vi "main_0510.vi"() -> ()   [LabVIEW 2018]
uses:
  <vilib>/Platform/TimedLoop/XDataNode/timing_clust.ctl
  <vilib>/Platform/TimedLoop/XDataNode/nitl_modes.ctl
  <vilib>/Platform/TimedLoop/XDataNode/wakeup.ctl
  <vilib>/FPGAPlugInAG/myRIO-1900/niLvFpga_Open_myRIO-1900.vi
  <vilib>/rvi/interface/common/dynamic/niFpgaDynamicAddResources.vi
  <vilib>/Utility/error.llb/Error Cluster From Error Code.vi
  <vilib>/rvi/errors/niLvFpgaAdjustHostInterfaceError.vi
  <vilib>/rvi/interface/nirviOpenFPGA/nirviOpenFPGA.xnode
  FPGA Bitfiles/Dentalrobot_FPGATarget_FPGADentalroboto_PTkoih3chUc.lvbitx
  FPGA/FPGA_myRIO.vi
  <vilib>/rvi/interface/nirviReadWriteControl/nirviReadWriteControl.xnode
  <vilib>/Platform/TimedLoop/XDataNode/XDataNode.xnode
  <vilib>/Platform/TimedLoop/XDataNode/XDNodeRunTimeDep.lvlib
  <vilib>/rvi/interface/Simulation/niFpgaSimulationCallBeginRW.vi
  NiFpgaLv.dll
panel:
  in  "Voltage Detect":bool
  in  "temp":i32
  in  "inverse(degree)":i32=90
  in  "limit_mV":u16=2000
  out "Finished Late":dbl
  in  "DIR4":bool
  out "Position4":i32
  in  "Reset 4":bool
  in  "STBY4":bool
  in  "ENA4":bool
  in  "CH4 DC":fxp<+,32,0>
  in  "RPM":string(combo)="150"
  in  "step":u32 step=2
  in  "Dir":bool=TRUE
  out "Voltage Detection (mV)":u16(graph)=459
  out "storeDC":fxp<+,32,0>[](array[numeric])
  in  "Inv":bool
  out "mV":u16
  in  "OK Button":bool
  out "position":i32[](array[numeric])
  out "Signal":bool[](array[boolean])
  out "Over Range":bool
  in  "stop":bool
  in  "Position":dbl step=1.0
  # "Servor"
  # "Stepper"
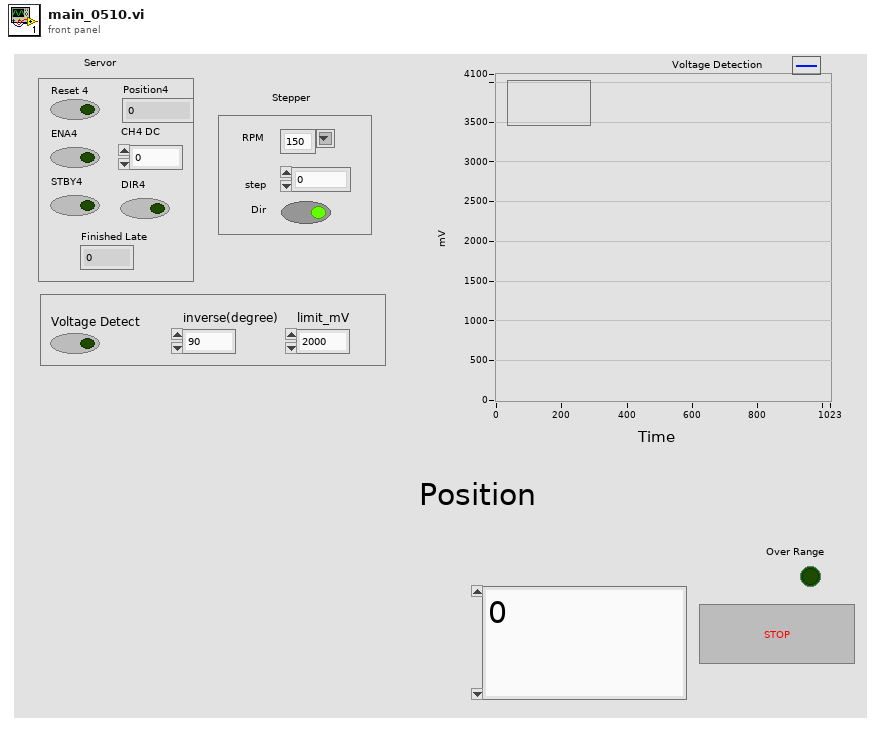
[diagram p1: front panel]
types:
  T1 = typedef "XDNodeRunTimeDep.lvlib/timing_clust.ctl" = cluster{"Expected End [f-1]":u64, "Actual End [f-1]":u64, "Finished Late? [f-1]":bool, "Expected End [i-1]":u64, "Actual End [i-1]":u64, "Finished Late? [i-1]":bool, "Expected Start [i]":u64, "Actual Start [i]":u64, "Expected Start [f]":u64, "Actual Start [f]":u64, "Source Name":string, "Structure Name":string, "Period":i64, "Deadline":i64, "Offset":i64, "Start":i64, "Priority":i32, "Timeout":i32, "Mode":T2, "Wakeup Reason":T3, "Error":errorcluster, "Source Type":string, "Secondary Source Type":string, "Global End Time":u64, "Global Start Time":u64, "Frame Duration":u64, "Iteration Duration":u64, "Assigned CPU":i32, "I/O Scan Engine Mode":u32}
  T2 = typedef "XDNodeRunTimeDep.lvlib/nitl_modes.ctl" = enum32{"No Change", "Process missed periods, maintain original phase", "Discard missed periods, maintain original phase", "Process missed periods, ignore original phase", "Discard missed periods, ignore original phase"}
  T3 = typedef "XDNodeRunTimeDep.lvlib/wakeup.ctl" = enum32{"Normal", "Aborted", "Asynchronous wakeup", "Timing source error", "Timed loop error", "Timeout"}
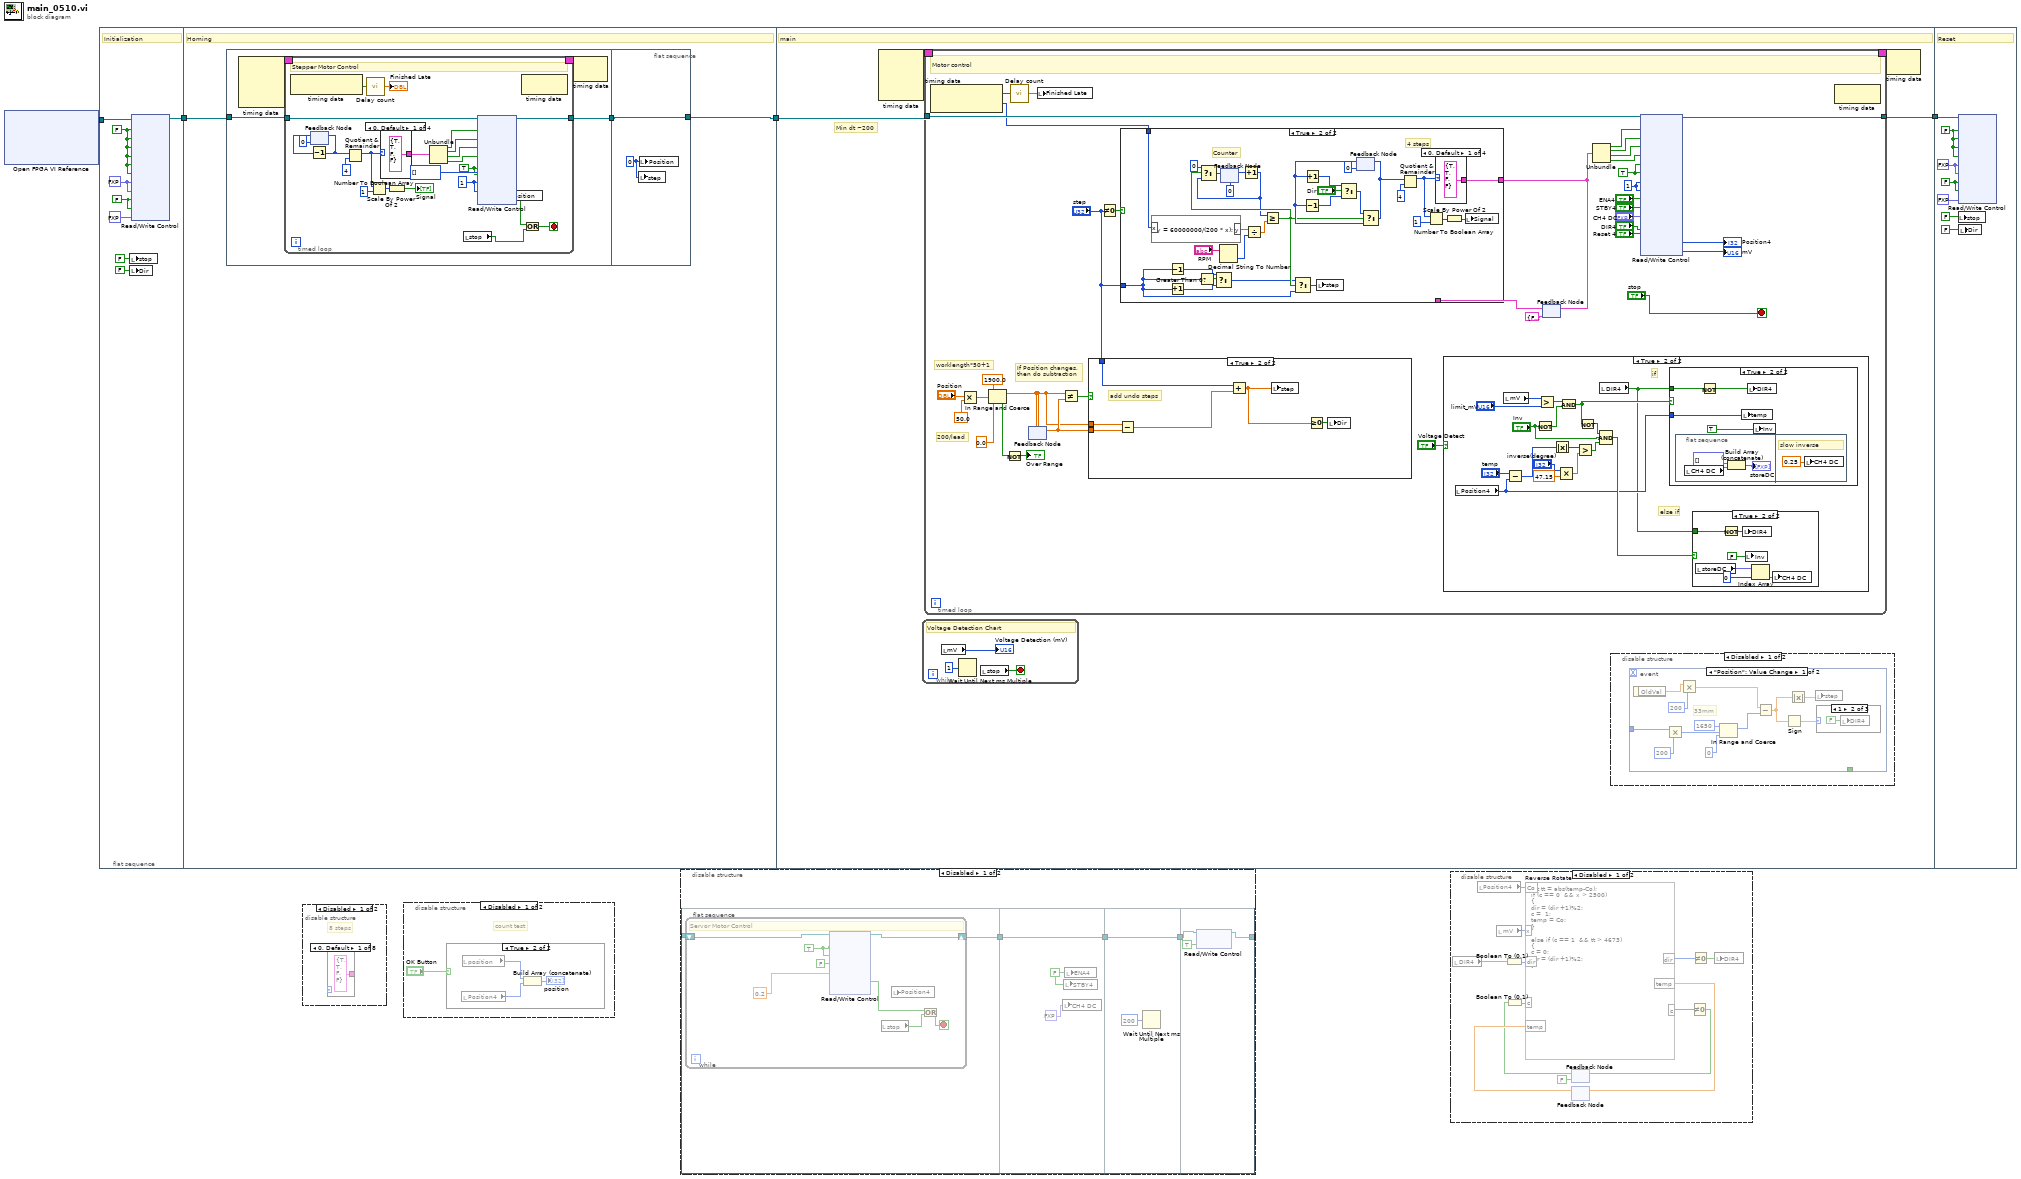
[diagram p0: block diagram]
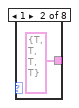
[diagram p6: hidden frame]
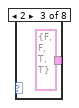
[diagram p7: hidden frame]
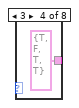
[diagram p8: hidden frame]
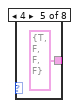
[diagram p9: hidden frame]
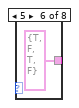
[diagram p10: hidden frame]
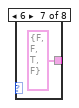
[diagram p11: hidden frame]
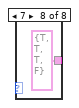
[diagram p12: hidden frame]
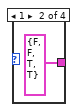
[diagram p14: hidden frame]
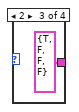
[diagram p15: hidden frame]
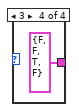
[diagram p16: hidden frame]
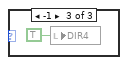
[diagram p18: hidden frame]
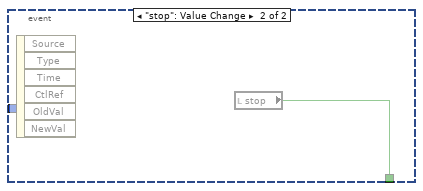
[diagram p19: hidden frame]
diagram:
  n1 = xnode "Open FPGA VI Reference"() -> ("FPGA VI Reference Out"=w1:refnum<k20>)  [unwired: 2 in, 1 out]
  n2 = flat-sequence {
    tunnel: [w11] -> w3
    tunnel: w1 -> [w9]
    tunnel: w3 -> [w14]
    tunnel: [w13] -> w2
    tunnel: [w57] -> w4
    tunnel: w2 -> [w56]
    tunnel: w4 -> [w195]
    frame #0 {
      w8 = FALSE ("ENA4")
      w10 = fxp<+,32,0> 0.0 ("CH1 DC")
      w12 = FALSE ("ENA1")
      # "Initialization"
      n3 = local write "stop"(FALSE ("stop")) -> ()
      n4 = local write "Dir"(FALSE ("Dir")) -> ()
      n5 = xnode "Read/Write Control"("FPGA VI Reference In"=w9, "ENA1"=w12, "STBY1"=w12, "DIR1"=w12, "ENA2"=w12, "STBY2"=w12, "DIR2"=w12, "CH1 DC"=w10, "CH2 DC"=w10, "ENA4"=w8, "STBY4"=w8, "CH4 DC"=fxp<+,32,0> 0.0) -> ("FPGA VI Reference Out"=w11:refnum<k20>)  [unwired: 1 in, 1 out]
    }
    frame #1 {
      # "Homing"
      n6 = flat-sequence {
        tunnel: [w17] -> w15
        tunnel: w14 -> [w16]
        tunnel: w15 -> [w53]
        tunnel: [w53] -> w13
        frame #0 {
          n7 = node-c288() -> (w20:T1)  [unwired: 4 in]
          n8 = timed-loop {
            timing: w20 -> [_]
            timing-out: [_] -> w19
            tunnel: w16 -> [w28]
            tunnel: [w27] -> w17
            stop <- w26 stop-if-true
            w41 = 1 ("CH1 DC")
            w42 = TRUE ("STBY1")
            # "Stepper Motor Control"
            n9 = node-c288() -> (w29:bool)  [unwired: 1 in]
            n10 = feedback #1(0) -> (w38:i32)
            n11 = Decrement(x=w38) -> (x-1=w30:i32)
            n12 = feedback-in #1(w30) -> ()
            n13 = Quotient & Remainder(x=w30, y=4) -> (x-y*floor(x/y)=w25:i32)  [unwired: 1 out]
            n14 = call "Delay count.vi"("Finished Late? [i-1]"=w29) -> ("Count"=→"Finished Late":dbl)
            n15 = Scale By Power Of 2(n=w25, x=u32 1) -> (x*2^n=w36:u32)
            n16 = case shown="0, Default" w25 {
              tunnel: [cluster{bool, bool, bool, bool} {TRUE, TRUE, FALSE, FALSE} cluster{bool, bool, bool, bool} {FALSE, FALSE, TRUE, TRUE} cluster{bool, bool, bool, bool} {TRUE, FALSE, FALSE, FALSE} cluster{bool, bool, bool, bool} {FALSE, FALSE, TRUE, FALSE}] -> w35
              frame 0, Default {
              }
              frame 1 {
              }
              frame 2 {
              }
              frame 3 {
              }
            }
            n17 = Number To Boolean Array(number=w36) -> (Boolean array=→"Signal":bool[])
            n18 = Unbundle(w35) -> (w34:bool, w33:bool, w32:bool, w31:bool)
            n19 = local read "stop"() -> (w22:bool)
            n20 = xnode "Read/Write Control"("FPGA VI Reference In"=w28, "ENA1"=w34, "DIR1"=w33, "ENA2"=w32, "DIR2"=w31, "STBY1"=w42, "STBY2"=w42, "CH1 DC"=w41, "CH2 DC"=w41) -> ("FPGA VI Reference Out"=w27:refnum<k20>, "C1"=w21:bool)  [unwired: 1 in, 1 out]
            n21 = node-c288() -> ()  [unwired: 1 in, 1 out]
            n22 = Or(x=w21, y=w22) -> (x .or. y?=w26:bool)
          }
          n23 = local write "position"(i32[] []) -> ()
          n24 = node-c288(w19) -> ()  [unwired: 1 out]
        }
        frame #1 {
          w52 = 0 ("Position")
          n25 = local write "step"(w52) -> ()
          n26 = local write "Position"(w52) -> ()
        }
      }
    }
    frame #2 {
      # "Min dt ~200"
      # "main"
      n27 = node-c288() -> (w55:T1)  [unwired: 4 in]
      n28 = while {
        stop <- w75 stop-if-true
        # "Voltage Detection Chart"
        n29 = local read "mV"() -> (→"Voltage Detection (mV)":u16)
        n30 = Wait Until Next ms Multiple(millisecond multiple=u32 1) -> ()  [unwired: 1 out]
        n31 = local read "stop"() -> (w75:bool)
      }
      n32 = timed-loop {
        timing: w55 -> [_]
        timing-out: [_] -> w54
        tunnel: [w110] -> w57
        tunnel: w56 -> [w109]
        stop <- "stop" stop-if-true
        w103 = 1 ("CH1 DC")
        w107 = TRUE ("STBY1")
        # "worklength*50+1"
        # "200/lead"
        # "If Position changes, \nthen do subtraction"
        # "Motor control"
        n33 = node-c288() -> (w94:bool, w95:i64)  [unwired: 1 in]
        n34 = Multiply(x="Position", y=50.0) -> (x*y=w78:dbl)
        n35 = In Range and Coerce(upper limit=1900.0, x=w78, lower limit=0.0) -> (coerced(x)=w82:dbl, In Range?=w81:bool)
        n36 = Not(x=w81) -> (.not. x?=→"Over Range":bool)
        n37 = call "Delay count.vi"("Finished Late? [i-1]"=w94) -> ("Count"=w93:dbl)
        n38 = feedback #2(w82) -> (w86:dbl)
        n39 = feedback-in #2(w82) -> ()
        n40 = local write "Finished Late"(w93) -> ()
        n41 = Not Equal?(x=w82, y=w86) -> (x != y?=w85:bool)
        n42 = case shown="True" w85 {
          tunnel: w86 -> [_ w115]
          tunnel: w82 -> [_ w116]
          tunnel: "step" -> [_ w111]
          frame False {
          }
          frame True {
            # "add undo steps"
            n43 = Subtract(x=w116, y=w115) -> (x-y=w114:dbl)
            n44 = Add(x=w111, y=w114) -> (x+y=w112:dbl)
            n45 = local write "step"(w112) -> ()
            n46 = Greater Or Equal To 0?(x=w112) -> (x >= 0?=w113:bool)
            n47 = local write "Dir"(w113) -> ()
          }
        }
        n48 = Not Equal To 0?(x="step") -> (x != 0?=w102:bool)
        n49 = case shown="True" "Voltage Detect" {
          frame False {
          }
          frame True {
            # "else if"
            # "if"
            n50 = local read "Position4"() -> (w123:i32)
            n51 = local read "mV"() -> (w125:u16)
            n52 = Subtract(x="temp", y=w123) -> (x-y=w129:i32)
            n53 = Not(x="Inv") -> (.not. x?=w132:bool)
            n54 = Greater?(x=w125, y="limit_mV") -> (0:w133:bool)
            n55 = Absolute Value(x=w129) -> (abs(x)=w119:i32)
            n56 = Multiply(x="inverse(degree)", y=47.15) -> (x*y=w118:dbl)
            n57 = And(x=w133, y=w132) -> (x .and. y?=w126:bool)
            n58 = Greater?(x=w119, y=w118) -> (0:w130:bool)
            n59 = Not(x=w126) -> (.not. x?=w131:bool)
            n60 = local read "DIR4"() -> (w117:bool)
            n61 = Compound Arithmetic op=AND(w131, "Inv", w130) -> (w127:bool)
            n62 = case shown="True" w126 {
              tunnel: w117 -> [_ w143]
              tunnel: w123 -> [_ w142]
              frame False {
              }
              frame True {
                n63 = flat-sequence {
                  frame #0 {
                    n64 = local read "CH4 DC"() -> (w144:fxp<+,32,0>)
                    n65 = Build Array (concatenate)(fxp<+,1,1>[] [], w144) -> (→"storeDC":fxp<+,32,0>[])
                  }
                  frame #1 {
                    # "slow inverse"
                    n66 = local write "CH4 DC"(0.25) -> ()
                  }
                }
                n67 = Not(x=w143) -> (.not. x?=w141:bool)
                n68 = local write "temp"(w142) -> ()
                n69 = local write "DIR4"(w141) -> ()
                n70 = local write "Inv"(TRUE ("Inv")) -> ()
              }
            }
            n71 = case shown="True" w127 {
              tunnel: w117 -> [_ w139]
              frame False {
              }
              frame True {
                n72 = local read "storeDC"() -> (w134:fxp<+,32,0>[])
                n73 = Not(x=w139) -> (.not. x?=w138:bool)
                n74 = local write "DIR4"(w138) -> ()
                n75 = local write "Inv"(FALSE ("Inv")) -> ()
                n76 = Index Array(array=w134, index=0) -> (element=w135:fxp<+,32,0>)
                n77 = local write "CH4 DC"(w135) -> ()
              }
            }
          }
        }
        n78 = feedback #3(cluster{bool, bool, bool, bool} {FALSE, FALSE, FALSE, FALSE}) -> (w101:cluster{bool, bool, bool, bool})
        n79 = case shown="True" w102 {
          tunnel: [w148 w178] -> w96
          tunnel: "step" -> [_ w149]
          tunnel: w101 -> [w148 _]
          tunnel: w95 -> [_ w156]
          frame False {
          }
          frame True {
            # "Counter"
            # "4 steps"
            # "convert  dt to rpm"
            n80 = formula code="y = 60000000/(200 * x);"("x"=w156) -> ("y"=w155:dbl)
            n81 = Decrement(x=w149) -> (x-1=w151:u32)
            n82 = Increment(x=w149) -> (x+1=w152:u32)
            n83 = Greater Than 0?(x=w149) -> (x > 0?=w153:bool)
            n84 = Select(t=w151, s=w153, f=w152) -> (s? t:f=w150:u32)
            n85 = Decimal String To Number(string="RPM") -> (number=w157:i32)  [unwired: 2 in, 1 out]
            n86 = feedback #4(0) -> (w167:i32)
            n87 = Increment(x=w167) -> (x+1=w166:i32)
            n88 = Divide(x=w155, y=w157) -> (x/y=w160:dbl)
            n89 = Greater Or Equal?(x=w166, y=w160) -> (x >= y?=w170:bool)
            n90 = Select(t=0, s=w170, f=w166) -> (s? t:f=w168:i32)
            n91 = feedback-in #4(w168) -> ()
            n92 = Select(t=w150, s=w170, f=w149) -> (s? t:f=w154:u32)
            n93 = local write "step"(w154) -> ()
            n94 = feedback #5(0) -> (w173:i32)
            n95 = Decrement(x=w173) -> (x-1=w172:i32)
            n96 = Increment(x=w173) -> (x+1=w174:i32)
            n97 = Select(t=w174, s="Dir", f=w172) -> (s? t:f=w171:i32)
            n98 = Select(t=w171, s=w170, f=w173) -> (s? t:f=w163:i32)
            n99 = feedback-in #5(w163) -> ()
            n100 = Quotient & Remainder(x=w163, y=4) -> (x-y*floor(x/y)=w159:i32)  [unwired: 1 out]
            n101 = Scale By Power Of 2(n=w159, x=u32 1) -> (x*2^n=w161:u32)
            n102 = case shown="0, Default" w159 {
              tunnel: [cluster{bool, bool, bool, bool} {TRUE, TRUE, FALSE, FALSE} cluster{bool, bool, bool, bool} {FALSE, FALSE, TRUE, TRUE} cluster{bool, bool, bool, bool} {TRUE, FALSE, FALSE, FALSE} cluster{bool, bool, bool, bool} {FALSE, FALSE, TRUE, FALSE}] -> w178
              frame 0, Default {
              }
              frame 1 {
              }
              frame 2 {
              }
              frame 3 {
              }
            }
            n103 = Number To Boolean Array(number=w161) -> (Boolean array=w158:bool[])
            n104 = local write "Signal"(w158) -> ()
          }
        }
        n105 = feedback-in #3(w96) -> ()
        n106 = Unbundle(w96) -> (w108:bool, w106:bool, w105:bool, w104:bool)
        n107 = xnode "Read/Write Control"("FPGA VI Reference In"=w109, "ENA1"=w108, "DIR1"=w106, "ENA2"=w105, "DIR2"=w104, "STBY1"=w107, "STBY2"=w107, "CH1 DC"=w103, "CH2 DC"=w103, "ENA4"="ENA4", "STBY4"="STBY4", "CH4 DC"="CH4 DC", "DIR4"="DIR4", "Reset 4"="Reset 4") -> ("FPGA VI Reference Out"=w110:refnum<k20>, "Position4"=→"Position4":i32, "Channel4"=→"mV":u16)  [unwired: 1 in, 1 out]
        n108 = node-c288() -> ()  [unwired: 1 in, 1 out]
      }
      n109 = disable-structure shown="Disabled" {
        frame Disabled {
          n110 = event shown="[0] \"Position\": Value Change" {
            selector: _ -> [_ _]
            dyn-events: _ -> [_ _]
            timeout: _ -> [_ _]
            tunnel: [_ w72] -> _
            tunnel: _ -> [w58 _]
            event "Position": Value Change {
              # "33mm"
              n111 = event-data() -> ("OldVal"=w60:dbl)  [unwired: 1 in]
              n112 = Multiply(x=w58, y=200) -> (x*y=w66:i32)
              n113 = Multiply(x=w60, y=200) -> (x*y=w59:dbl)
              n114 = In Range and Coerce(upper limit=1650, x=w66, lower limit=0 ("x")) -> (coerced(x)=w67:i32)  [unwired: 1 out]
              n115 = Subtract(x=w59, y=w67) -> (x-y=w64:dbl)
              n116 = Sign(1:w64) -> (0:w63:dbl)
              n117 = Absolute Value(x=w64) -> (abs(x)=w62:dbl)
              n118 = local write "step"(w62) -> ()
              n119 = case shown="1" w63 {
                frame 0, Default {
                }
                frame 1 {
                  n120 = local write "DIR4"(FALSE ("DIR4")) -> ()
                }
                frame -1 {
                  n121 = local write "DIR4"(TRUE ("DIR4")) -> ()
                }
              }
            }
            event "stop": Value Change {
              n122 = event-data() -> ()  [unwired: 1 in, 6 out]
              n123 = local read "stop"() -> (w72:bool)
            }
          }
        }
        frame Enabled {
        }
      }
      n124 = node-c288(w54) -> ()  [unwired: 1 out]
    }
    frame #3 {
      w192 = FALSE ("ENA4")
      w193 = fxp<+,32,0> 0.0 ("CH1 DC")
      w194 = FALSE ("ENA1")
      # "Reset"
      n125 = xnode "Read/Write Control"("FPGA VI Reference In"=w195, "ENA1"=w194, "STBY1"=w194, "ENA2"=w194, "STBY2"=w194, "CH1 DC"=w193, "CH2 DC"=w193, "ENA4"=w192, "STBY4"=w192, "CH4 DC"=fxp<+,32,0> 0.0) -> ()  [unwired: 1 in, 2 out]
      n126 = local write "stop"(FALSE ("stop")) -> ()
      n127 = local write "Dir"(FALSE ("Dir")) -> ()
    }
  }
  n128 = disable-structure shown="Disabled" {
    frame Disabled {
      # "8 steps"
      n129 = case shown="0, Default" {
        selector: _ -> [_ _ w199 _ _ _ _ _]
        tunnel: [cluster{bool, bool, bool, bool} {TRUE, TRUE, FALSE, FALSE} cluster{bool, bool, bool, bool} {TRUE, TRUE, TRUE, TRUE} cluster{bool, bool, bool, bool} {FALSE, FALSE, TRUE, TRUE} cluster{bool, bool, bool, bool} {TRUE, FALSE, TRUE, TRUE} cluster{bool, bool, bool, bool} {TRUE, FALSE, FALSE, FALSE} cluster{bool, bool, bool, bool} {TRUE, FALSE, TRUE, FALSE} cluster{bool, bool, bool, bool} {FALSE, FALSE, TRUE, FALSE} cluster{bool, bool, bool, bool} {TRUE, TRUE, TRUE, FALSE}] -> _
        frame 0, Default {
        }
        frame 1 {
        }
        frame 2 {
        }
        frame 3 {
        }
        frame 4 {
        }
        frame 5 {
        }
        frame 6 {
        }
        frame 7 {
        }
      }
    }
    frame Enabled {
    }
  }
  n130 = disable-structure shown="Disabled" {
    frame Disabled {
      # "count test"
      n131 = case shown="True" "OK Button" {
        frame False {
        }
        frame True {
          n132 = local read "Position4"() -> (w207:i32)
          n133 = local read "position"() -> (w208:i32[])
          n134 = Build Array (concatenate)(w208, w207) -> (→"position":i32[])
        }
      }
    }
    frame Enabled {
    }
  }
  n135 = disable-structure shown="Disabled" {
    disable-tunnel: [w209 _] -> _
    frame Disabled {
      n136 = flat-sequence {
        tunnel: _ -> [w214]
        tunnel: [w213] -> w212
        tunnel: w212 -> [w226]
        tunnel: [w226] -> w211
        tunnel: w211 -> [w228]
        tunnel: [w228] -> w210
        tunnel: [w229] -> w209
        tunnel: w210 -> [w231]
        frame #0 {
          n137 = while {
            shift-right: [w222] -> w213
            shift-left: w214 -> [w223]
            stop <- w219 stop-if-true
            w221 = TRUE ("ENA4")
            # "Servor Motor Control"
            n138 = xnode "Read/Write Control"("FPGA VI Reference In"=w223, "ENA4"=w221, "STBY4"=w221, "DIR4"=FALSE, "CH4 DC"=0.2) -> ("FPGA VI Reference Out"=w222:refnum<k20>, "C1"=w215:bool, "Position4"=w216:i32)  [unwired: 1 in, 1 out]
            n139 = local read "stop"() -> (w217:bool)
            n140 = local read "Position4"() -> ()  [unwired: 1 in]
            n141 = Or(x=w215, y=w217) -> (x .or. y?=w219:bool)
          }
        }
        frame #1 {
          w225 = FALSE ("ENA4")
          n142 = local write "CH4 DC"(fxp<+,32,0> 0.0 ("CH4 DC")) -> ()
          n143 = local write "STBY4"(w225) -> ()
          n144 = local write "ENA4"(w225) -> ()
        }
        frame #2 {
          n145 = Wait Until Next ms Multiple(millisecond multiple=u32 200) -> ()  [unwired: 1 out]
        }
        frame #3 {
          n146 = xnode "Read/Write Control"("FPGA VI Reference In"=w231, "Reset 4"=TRUE) -> ("FPGA VI Reference Out"=w229:refnum<k20>)  [unwired: 1 in, 1 out]
        }
      }
    }
    frame Enabled {
    }
  }
  n147 = disable-structure shown="Disabled" {
    frame Disabled {
      n148 = local read "DIR4"() -> (w244:bool)
      n149 = local read "Position4"() -> (w242:i32)
      n150 = local read "mV"() -> (w241:u16)
      n151 = Boolean To (0,1)(Boolean=w244) -> (0, 1=w232:i16)
      n152 = feedback #6() -> (w240:dbl)  [unwired: 1 in]
      n153 = feedback #7(FALSE) -> (w237:bool)
      n154 = Boolean To (0,1)(Boolean=w237) -> (0, 1=w235:i16)
      n155 = formula code="int tt = abs(temp-Co);\nif (c == 0  && x > 2500)\n{\ndir = (dir +1)%2;\nc =  1;\ntemp = Co;\n}\n\nelse if (c == 1  && tt > 4673)\n{\nc = 0;\ndir = (dir +1)%2;\n}" "Reverse Rotate"("x"=w241, "dir"=w232, "c"=w235, "Co"=w242, "temp"=w240) -> ("dir"=w233:i16, "c"=w234:i16, "temp"=w239:dbl)
      n156 = feedback-in #6(w239) -> ()
      n157 = Not Equal To 0?(x=w234) -> (x != 0?=w236:bool)
      n158 = feedback-in #7(w236) -> ()
      n159 = Not Equal To 0?(x=w233) -> (x != 0?=w243:bool)
      n160 = local write "DIR4"(w243) -> ()
    }
    frame Enabled {
    }
  }
